vi "main.vi"() -> ()   [LabVIEW 2026]
uses:
  Controller Commands.ctl
  5a459cdc-f68a-1c45-a763-c7efc7f6e060.vi
  <vilib>/Utility/error.llb/Trim Whitespace (string).vi
  <vilib>/Utility/error.llb/Trim Whitespace One-Sided.vi
  <vilib>/Instr/_visa.llb/VISA Configure Serial Port (Instr).vi
panel:
  in  "Find Curriculum":bool
  in  "Plot to graph":bool
  in  "Reads":i32
  in  "Patameters":string[](array[string])
  in  "Command":string
  in  "Device Commands":i32(listbox)
  in  "Send Command":bool
  in  "Run Example":bool
  in  "See commands":bool
  in  "Connected Devices":i32(listbox)
  in  "Search for devices":bool
  in  "About":string="  About this app"
  in  "Status Messages":string
  in  "Exit Program":bool
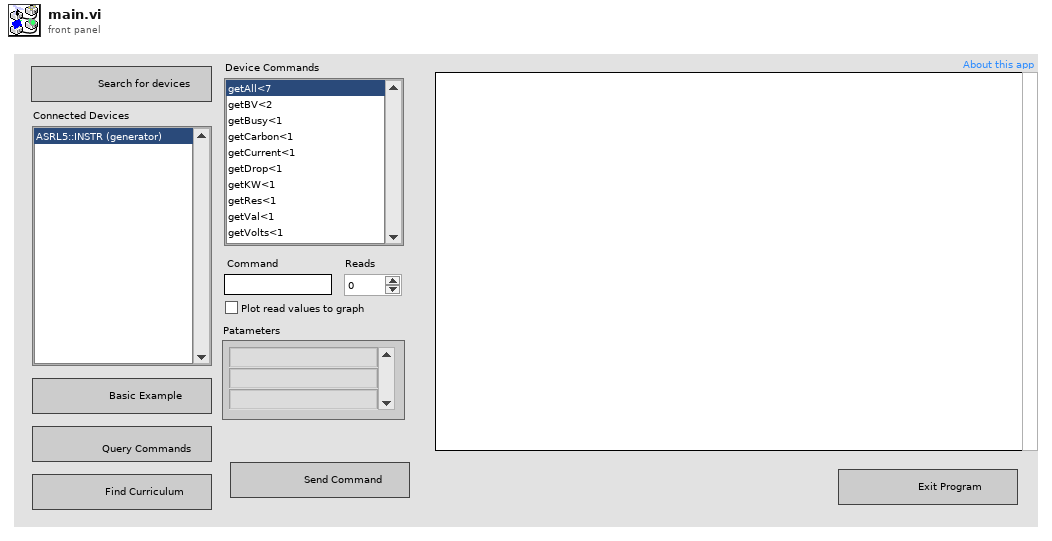
[diagram p1: front panel]
types:
  T1 = typedef "Controller Commands.ctl" = cluster{"Command":enum16{"Request Commands", "Clear all VISA aliases", "Read Reply", "Display Commands", "Command Selected", "Update UI", "Send Command", "Initialize UI", "Device Highlighted", "Run Example", "Detect Devices", "End Program", "Example Finder", "Retrieve Commands"}, "Variant":variant}
  T2 = cluster{"Connected Devices":refnum<vi>, "Device type":string[], "VISA Aliases":string[], "Status Messages":refnum<vi>, "Run Example":refnum<vi>, "See commands":refnum<vi>, "Array of VISA Resources":refnum<visa-resource-name>[], "Map of Commands":map{string, set{string}}, "Device Commands":refnum<vi>, "Command":refnum<vi>, "Patameters":refnum<vi>, "Reads":refnum<vi>, "queue for graph":refnum<queue>, "Send Command":refnum<vi>, "Find Curriculum":refnum<vi>, "appended path":path}
  T3 = enum8{"Enabled", "Disabled", "Disabled and Grayed Out"}
  T4 = enum32{"Invalid", "Standard", "Closed", "Hidden", "Minimized", "Maximized"}
  T5 = cluster{"Devices":i32, "Selected Command":string}
  T6 = enum16{"Request Commands", "Clear all VISA aliases", "Read Reply", "Display Commands", "Command Selected", "Update UI", "Send Command", "Initialize UI", "Device Highlighted", "Run Example", "Detect Devices", "End Program", "Example Finder", "Retrieve Commands"}
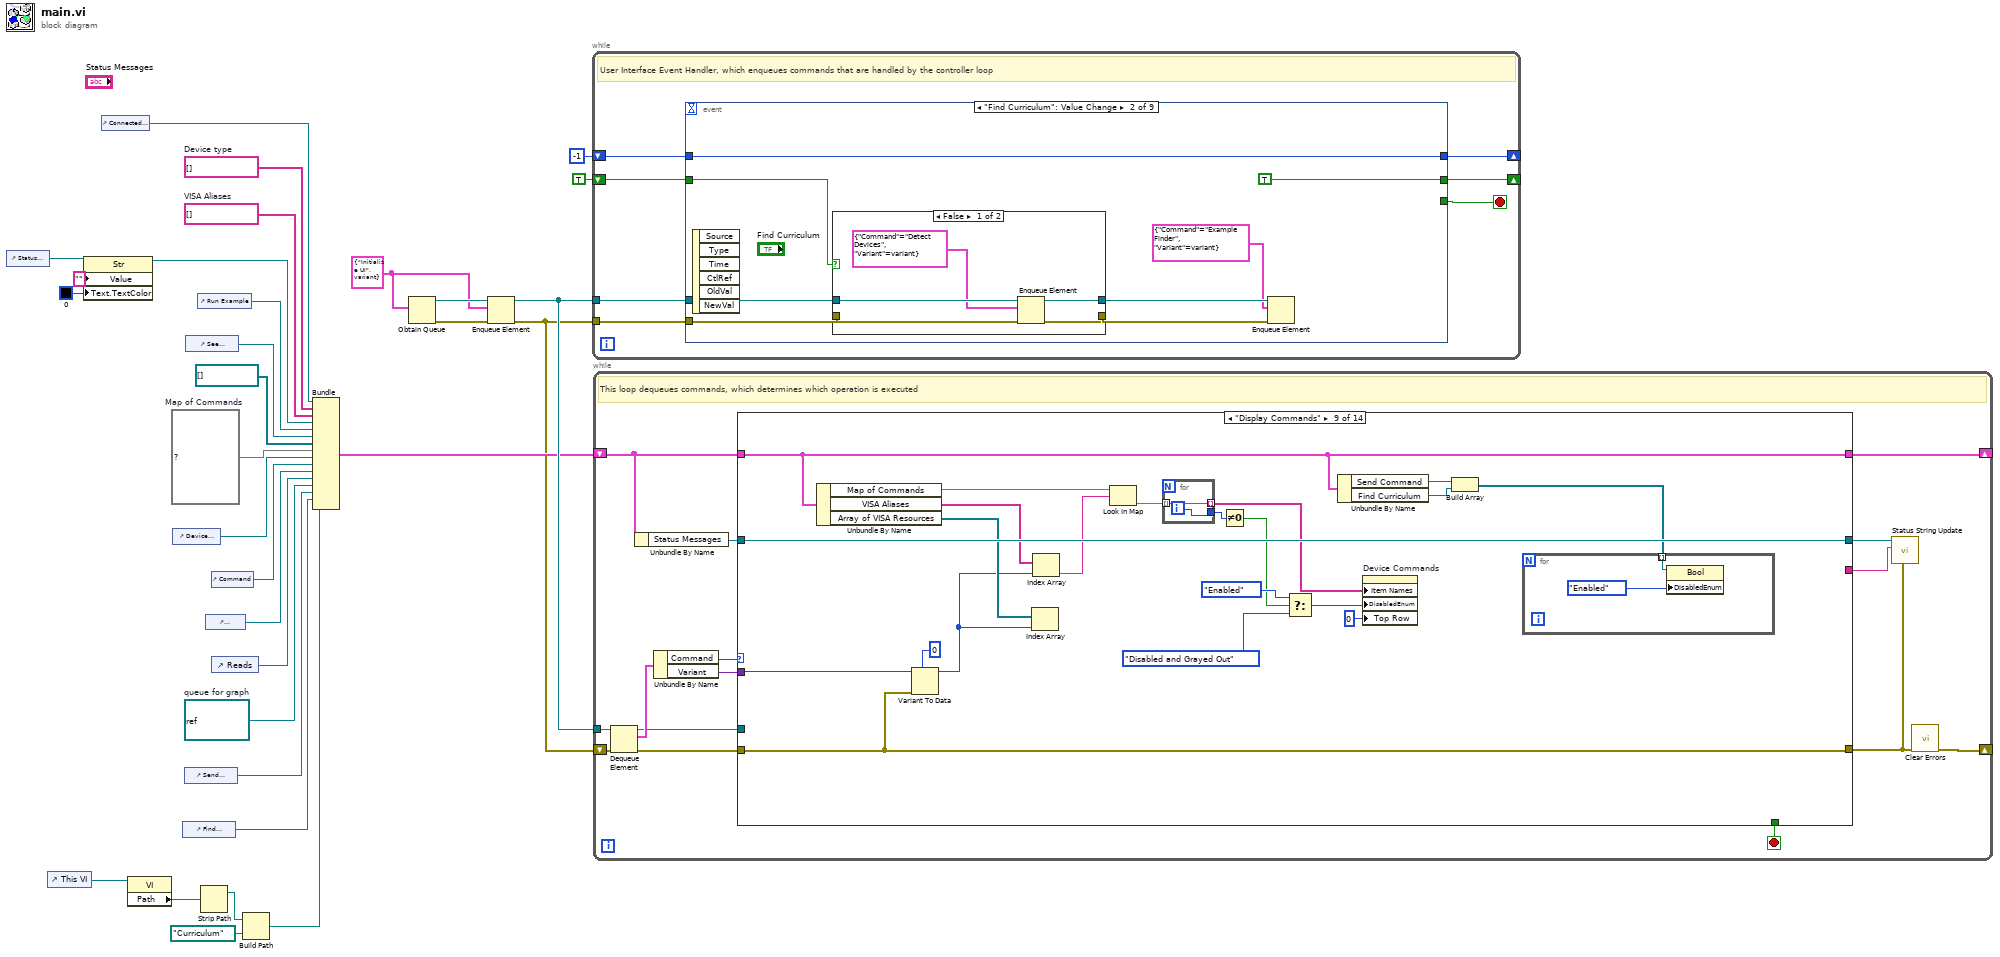
[diagram p0: block diagram]
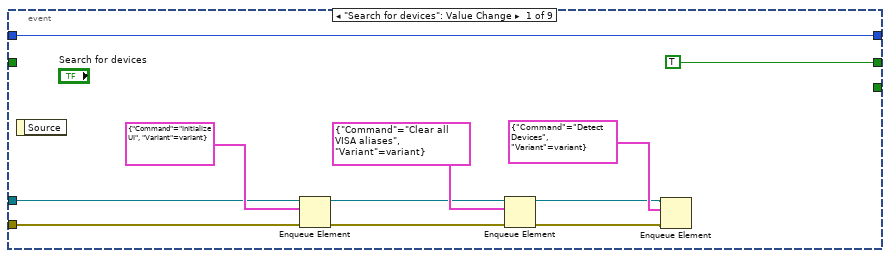
[diagram p2: hidden frame]
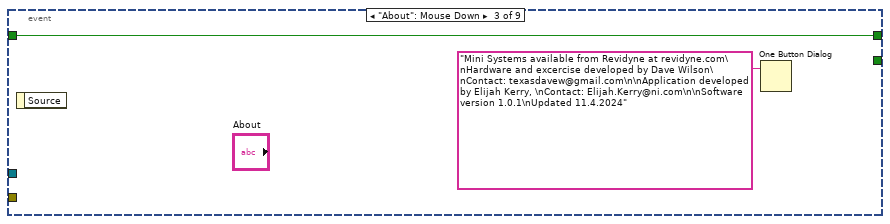
[diagram p4: hidden frame]
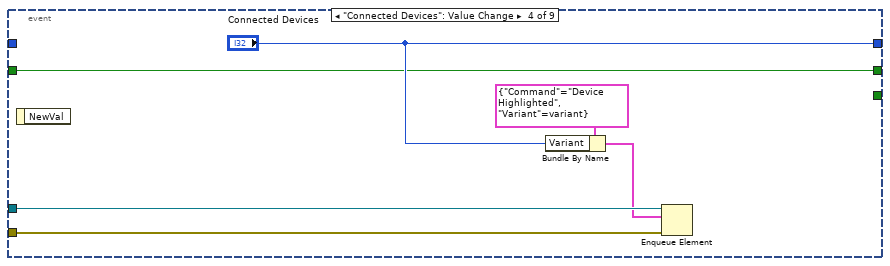
[diagram p5: hidden frame]
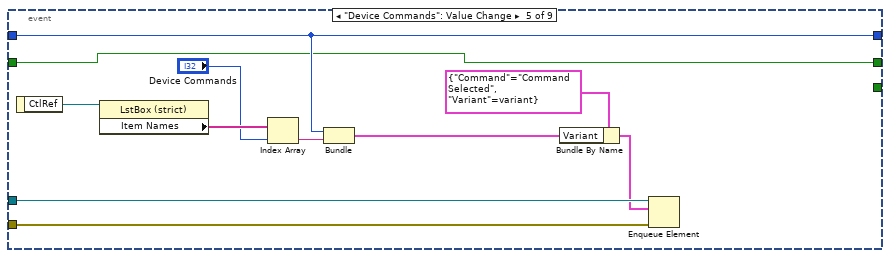
[diagram p6: hidden frame]
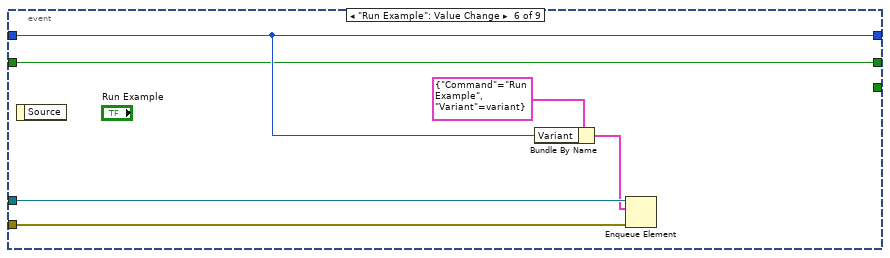
[diagram p7: hidden frame]
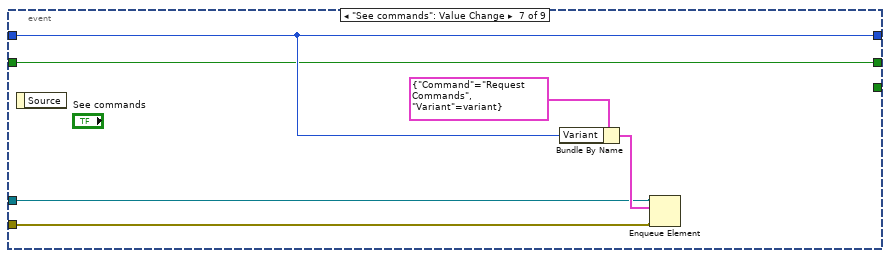
[diagram p8: hidden frame]
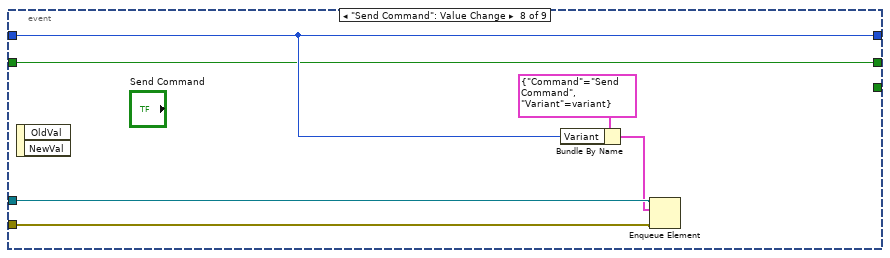
[diagram p9: hidden frame]
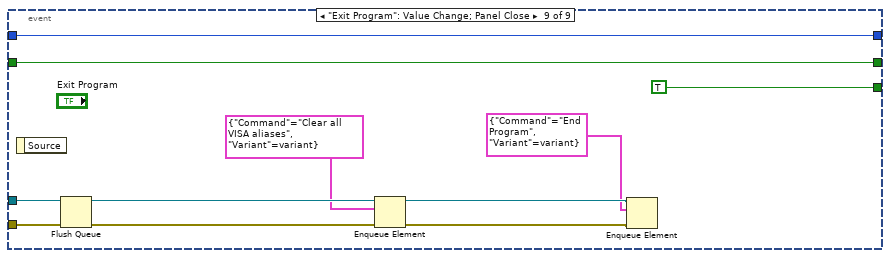
[diagram p10: hidden frame]
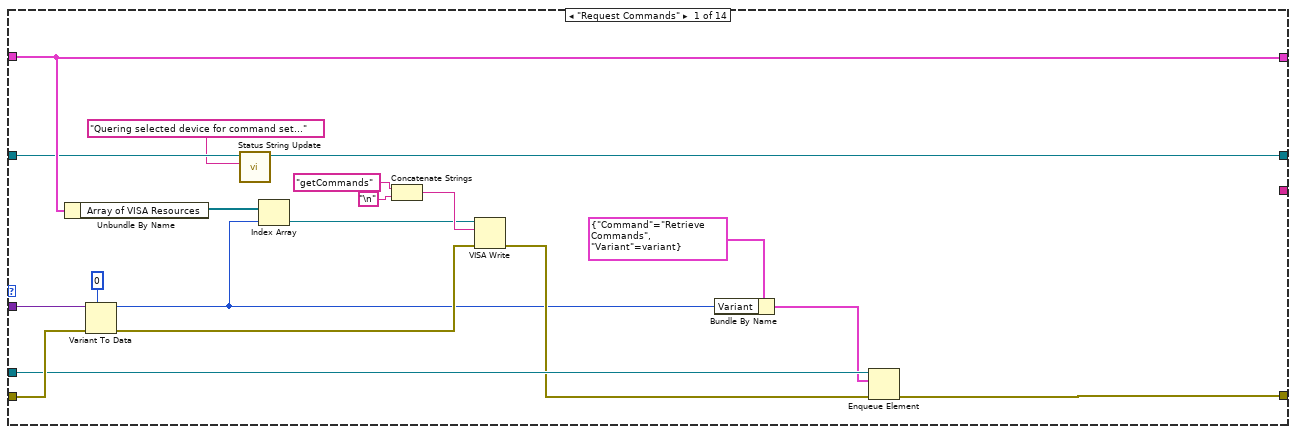
[diagram p11: hidden frame]
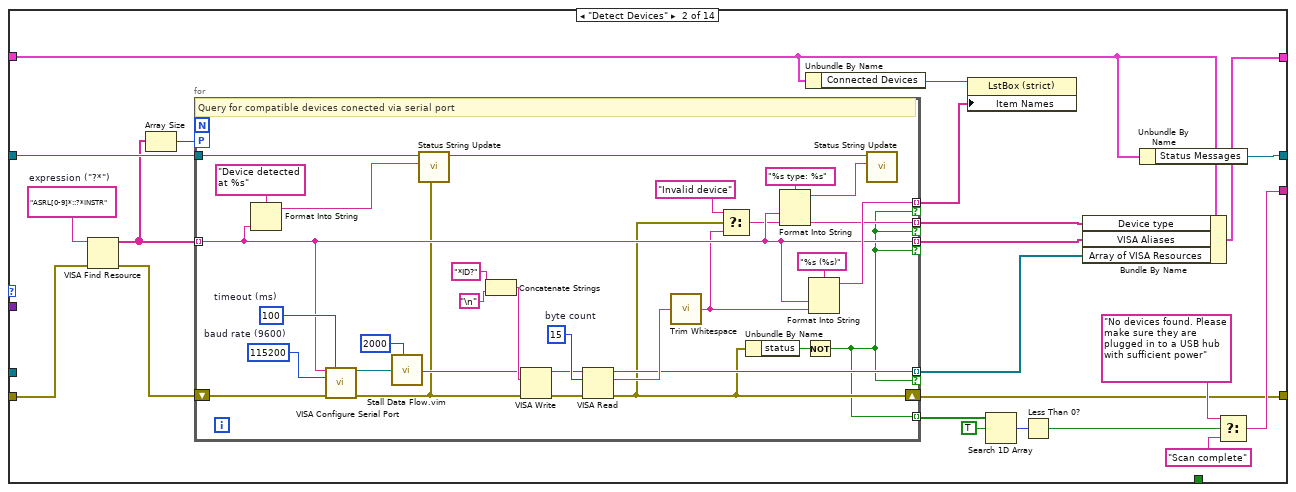
[diagram p12: hidden frame]
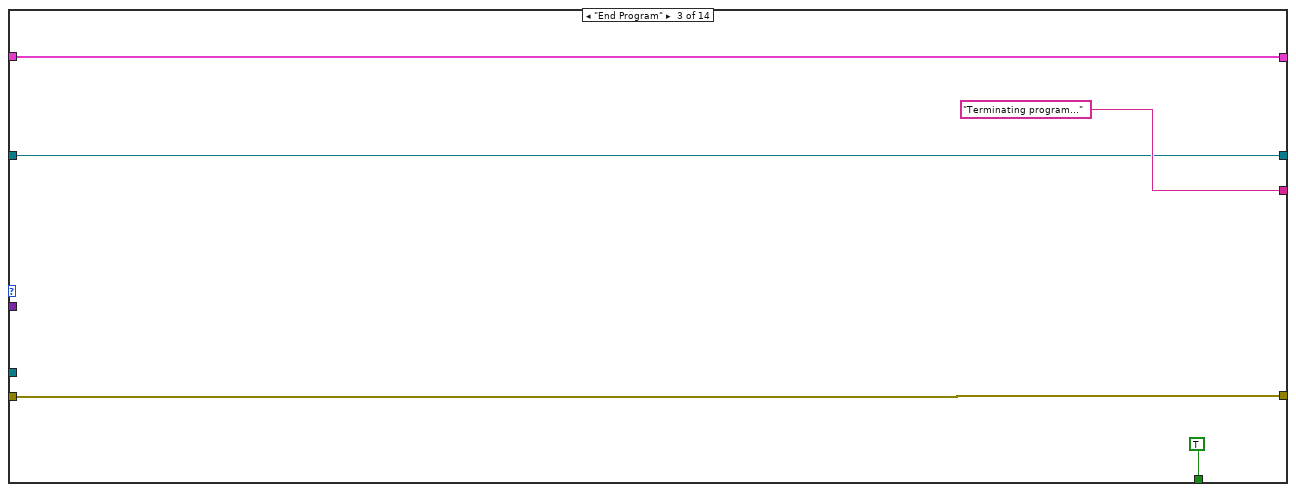
[diagram p13: hidden frame]
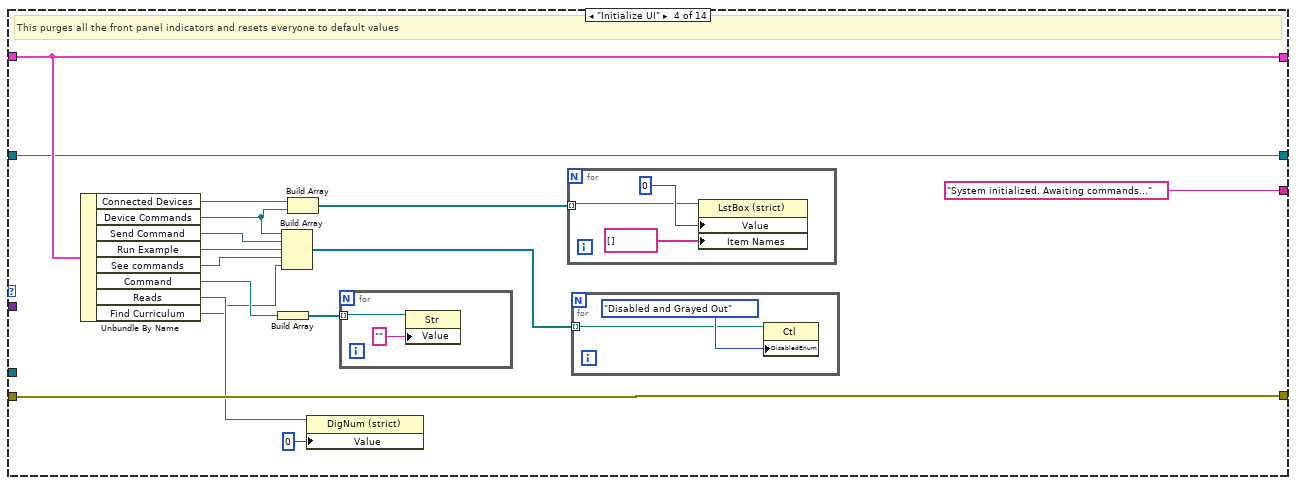
[diagram p14: hidden frame]
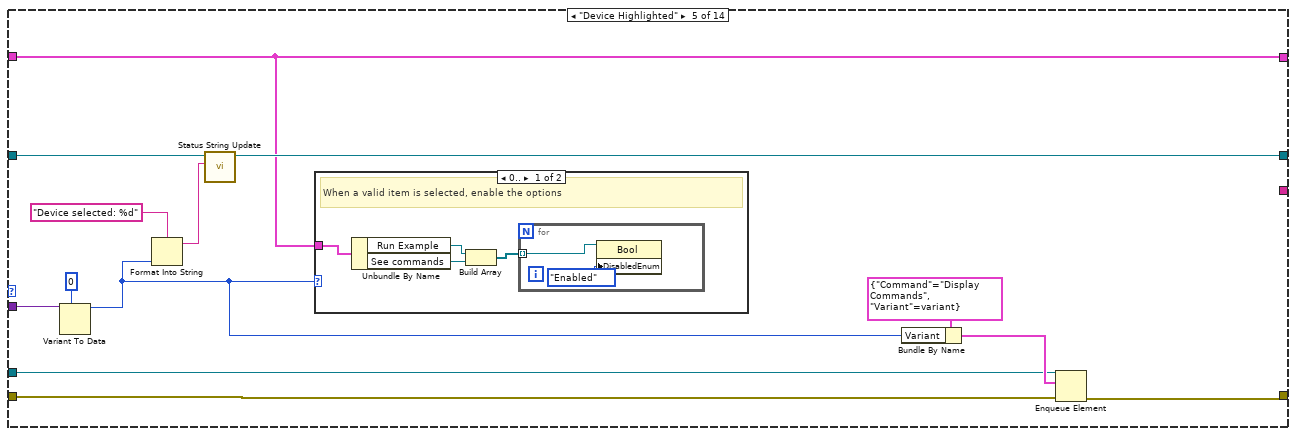
[diagram p15: hidden frame]
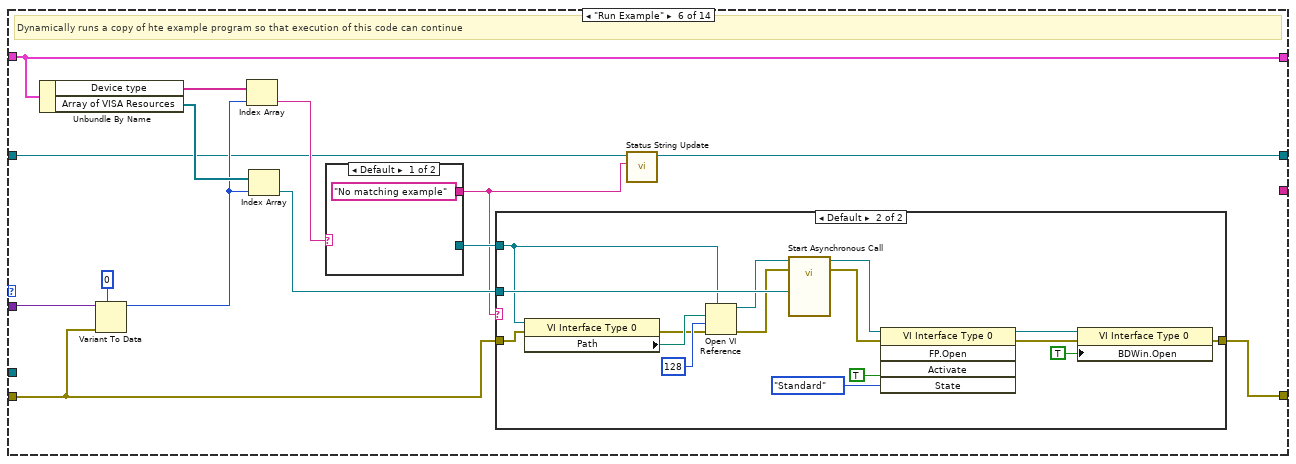
[diagram p17: hidden frame]
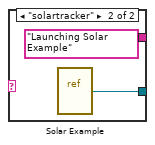
[diagram p19: hidden frame]
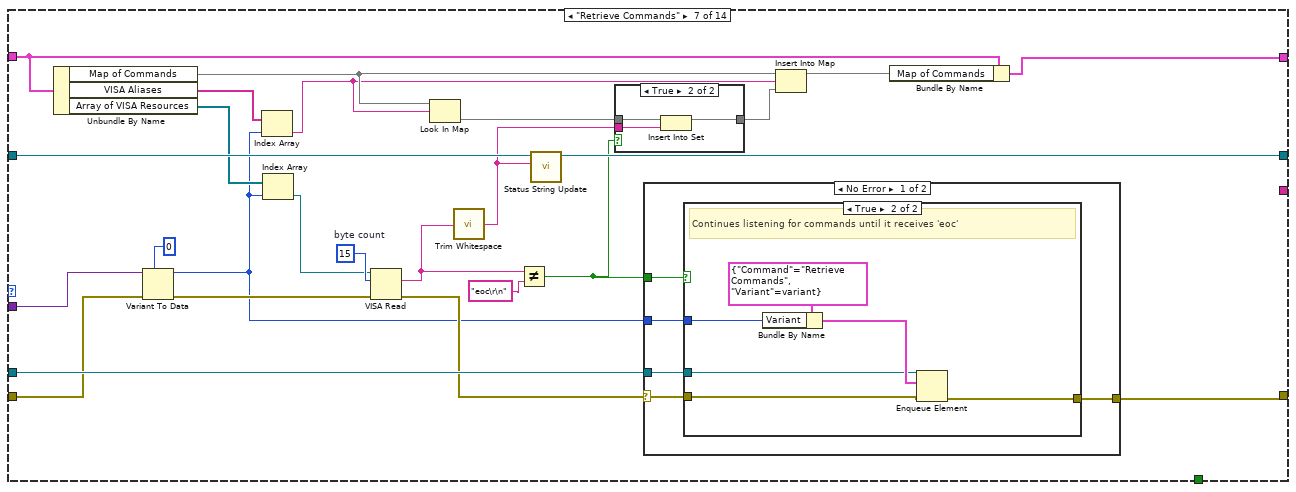
[diagram p20: hidden frame]
diagram:
  w13 = refnum<queue> refnum  # queue for graph
  w18 = map{string, set{string}} {}  # Map of Commands
  w19 = string[] []  # Device type
  w27 = string[] []  # VISA Aliases
  w29 = T1 {"Command"=enum."Initialize UI", "Variant"=variant} ("Controller Commands")
  n1 = control-ref of="Status Messages"() -> (w11:refnum<vi>)
  n2 = control-ref of="This VI"() -> (w4:refnum<vi>)
  n3 = property on="Property Node" class="Str"(reference=w11, "Value"="", "Text.TextColor"=u32 0 ("Text.Text Colors:Text Color")) -> (reference out=w10:refnum<vi>)  [unwired: 1 in, 1 out]
  n4 = control-ref of="Connected Devices"() -> (w20:refnum<vi>)
  n5 = property class="VI"(reference=w4) -> ("Path"=w5:path)  [unwired: 1 in, 2 out]
  n6 = control-ref of="Device Commands"() -> (w17:refnum<vi>)
  n7 = control-ref of="Find Curriculum"() -> (w7:refnum<vi>)
  n8 = control-ref of="Send Command"() -> (w12:refnum<vi>)
  n9 = control-ref of="See commands"() -> (w24:refnum<vi>)
  n10 = control-ref of="Run Example"() -> (w25:refnum<vi>)
  n11 = Strip Path(path=w5) -> (stripped path=w6:path)  [unwired: 1 out]
  n12 = control-ref of="Patameters"() -> (w15:refnum<vi>)
  n13 = control-ref of="Command"() -> (w16:refnum<vi>)
  n14 = control-ref of="Reads"() -> (w14:refnum<vi>)
  n15 = Build Path(base path=w6, name or relative path=path "Curriculum") -> (appended path=w2:path)
  n16 = Bundle("Connected Devices"=w20, "Device type"=w19, "VISA Aliases"=w27, "Status Messages"=w10, "Run Example"=w25, "See commands"=w24, "Array of VISA Resources"=refnum<visa-resource-name>[] [], "Map of Commands"=w18, "Device Commands"=w17, "Command"=w16, "Patameters"=w15, "Reads"=w14, "queue for graph"=w13, "Send Command"=w12, "Find Curriculum"=w7, "appended path"=w2) -> (w26:T2)  [unwired: 1 in]
  n17 = Obtain Queue(element data type=w29) -> (queue out=w31:refnum<queue>, error out=w28:errorcluster)  [unwired: 4 in, 1 out]
  n18 = Enqueue Element(queue=w31, element=w29, error in (no error)=w28) -> (queue out=w30:refnum<queue>, error out=w23:errorcluster)  [unwired: 1 in, 1 out]
  n19 = while {
    tunnel: w30 -> [w35]
    tunnel: w23 -> [w34]
    shift-right: [w37] -> _
    shift-left: -1 ("Connected Devices") -> [w36]
    shift-right: [w32] -> _
    shift-left: TRUE ("Find Curriculum") -> [w33]
    stop <- w38 stop-if-true
    # "User Interface Event Handler, which enqueues commands that are handled by the controller loop"
    n20 = event shown="[1] \"Find Curriculum\": Value Change" {
      selector: _ -> [_ _ _ _ _ _ _ _ _]
      dyn-events: _ -> [_ _ _ _ _ _ _ _ _]
      timeout: _ -> [_ _ _ _ _ _ _ _ _]
      tunnel: [_ _ _ _ _ _ _ _ TRUE] -> w38
      tunnel: w36 -> [w49 w55 _ _ w78 w88 w94 w100 w111]
      tunnel: [w49 w55 _ "Connected Devices" w78 w88 w94 w100 w111] -> w37
      tunnel: w35 -> [w44 w57 _ w69 w75 w86 w91 w98 w110]
      tunnel: w34 -> [w43 w56 _ w68 w74 w85 w90 w96 w109]
      tunnel: w33 -> [_ w54 w66 w70 w76 w87 w93 w99 w105]
      tunnel: [TRUE ("Find Curriculum") TRUE ("Find Curriculum") w66 w70 w76 w87 w93 w99 w105] -> w32
      event "Search for devices": Value Change {
        n21 = event-data() -> ()  [unwired: 1 in, 1 out]
        n22 = Enqueue Element(queue=w44, element=T1 {"Command"=enum."Initialize UI", "Variant"=variant}, error in (no error)=w43) -> (queue out=w45:refnum<queue>, error out=w46:errorcluster)  [unwired: 1 in, 1 out]
        n23 = Enqueue Element(queue=w45, element=T1 {"Command"=enum."Clear all VISA aliases", "Variant"=variant}, error in (no error)=w46) -> (queue out=w40:refnum<queue>, error out=w39:errorcluster)  [unwired: 1 in, 1 out]
        n24 = Enqueue Element(queue=w40, element=T1 {"Command"=enum."Detect Devices", "Variant"=variant}, error in (no error)=w39) -> ()  [unwired: 1 in, 3 out]
      }
      event "Find Curriculum": Value Change {
        n25 = event-data() -> ()  [unwired: 1 in, 6 out]
        n26 = case shown="False" w54 {
          tunnel: w57 -> [w62 w64]
          tunnel: [w61 w64] -> w52
          tunnel: w56 -> [w60 w63]
          tunnel: [w59 w63] -> w51
          frame False {
            n27 = Enqueue Element(queue=w62, element=T1 {"Command"=enum."Detect Devices", "Variant"=variant}, error in (no error)=w60) -> (queue out=w61:refnum<queue>, error out=w59:errorcluster)  [unwired: 1 in, 1 out]
          }
          frame True {
          }
        }
        n28 = Enqueue Element(queue=w52, element=T1 {"Command"=enum."Example Finder", "Variant"=variant}, error in (no error)=w51) -> ()  [unwired: 1 in, 3 out]
      }
      event "About": Mouse Down {
        n29 = event-data() -> ()  [unwired: 1 in, 1 out]
        n30 = One Button Dialog(message="Mini Systems available from Revidyne at revidyne.com\nHardware and excercise developed by Dave Wilson\nContact: texasdavew@gmail.com\n\nApplication developed by Elijah Kerry, \nContact: Elijah.Kerry@ni.com\n\nSoftware version 1.0.1\nUpdated 11.4.2024") -> ()  [unwired: 1 in, 1 out]
      }
      event "Connected Devices": Value Change {
        n31 = event-data() -> ()  [unwired: 1 in, 1 out]
        n32 = Bundle By Name(cluster=T1 {"Command"=enum."Device Highlighted", "Variant"=variant} ("Controller Commands"), "Variant"="Connected Devices") -> (w67:T1)
        n33 = Enqueue Element(queue=w69, element=w67, error in (no error)=w68) -> ()  [unwired: 1 in, 3 out]
      }
      event "Device Commands": Value Change {
        n34 = event-data() -> ("CtlRef"=w82:refnum<vi>)  [unwired: 1 in]
        n35 = property class="LstBox (strict)"(reference=w82) -> ("Item Names"=w81:string[])  [unwired: 1 in, 2 out]
        n36 = Index Array(array=w81, index="Device Commands") -> (element=w77:string)
        n37 = Bundle("Connected Devices"=w78, w77) -> (w79:cluster{"Connected Devices":i32, string})  [unwired: 1 in]
        n38 = Bundle By Name(cluster=T1 {"Command"=enum."Command Selected", "Variant"=variant} ("Controller Commands"), "Variant"=w79) -> (w73:T1)
        n39 = Enqueue Element(queue=w75, element=w73, error in (no error)=w74) -> ()  [unwired: 1 in, 3 out]
      }
      event "Run Example": Value Change {
        n40 = event-data() -> ()  [unwired: 1 in, 1 out]
        n41 = Bundle By Name(cluster=T1 {"Command"=enum."Run Example", "Variant"=variant} ("Controller Commands"), "Variant"=w88) -> (w84:T1)
        n42 = Enqueue Element(queue=w86, element=w84, error in (no error)=w85) -> ()  [unwired: 1 in, 3 out]
      }
      event "See commands": Value Change {
        n43 = event-data() -> ()  [unwired: 1 in, 1 out]
        n44 = Bundle By Name(cluster=T1 {"Command"=enum."Request Commands", "Variant"=variant} ("Controller Commands"), "Variant"=w94) -> (w92:T1)
        n45 = Enqueue Element(queue=w91, element=w92, error in (no error)=w90) -> ()  [unwired: 1 in, 3 out]
      }
      event "Send Command": Value Change {
        n46 = event-data() -> ()  [unwired: 1 in, 2 out]
        n47 = Bundle By Name(cluster=T1 {"Command"=enum."Send Command", "Variant"=variant} ("Controller Commands"), "Variant"=w100) -> (w97:T1)
        n48 = Enqueue Element(queue=w98, element=w97, error in (no error)=w96) -> ()  [unwired: 1 in, 3 out]
      }
      event "Exit Program": Value Change; Panel Close {
        n49 = event-data() -> ()  [unwired: 1 in, 1 out]
        n50 = Flush Queue(queue=w110, error in (no error)=w109) -> (queue out=w107:refnum<queue>, error out=w108:errorcluster)  [unwired: 1 out]
        n51 = Enqueue Element(queue=w107, element=T1 {"Command"=enum."Clear all VISA aliases", "Variant"=variant}, error in (no error)=w108) -> (queue out=w104:refnum<queue>, error out=w103:errorcluster)  [unwired: 1 in, 1 out]
        n52 = Enqueue Element(queue=w104, element=T1 {"Command"=enum."End Program", "Variant"=variant}, error in (no error)=w103) -> ()  [unwired: 1 in, 3 out]
      }
    }
  }
  n53 = while {
    shift-right: [w122] -> _
    shift-left: w26 -> [w120]
    tunnel: w30 -> [w127]
    shift-right: [w115] -> _
    shift-left: w23 -> [w124]
    stop <- w116 stop-if-true
    # "This loop dequeues commands, which determines which operation is executed"
    n54 = Dequeue Element(queue=w127, error in (no error)=w124) -> (queue out=w114:refnum<queue>, element=w126:T1, error out=w123:errorcluster)  [unwired: 1 in, 1 out]
    n55 = Unbundle By Name(w120) -> ("Status Messages"=w119:refnum<vi>)
    n56 = Unbundle By Name(w126) -> ("Command"=w125:T6, "Variant"=w117:variant)
    n57 = case shown="\"Display Commands\"" w125 {
      tunnel: [_ _ TRUE _ _ _ _ _ _ _ _ _ _ _] -> w116
      tunnel: w120 -> [w144 w149 w200 w219 w235 w255 w289 w329 w334 w361 w410 w448 w469 w485]
      tunnel: w123 -> [w134 w167 w199 w216 w230 w251 w298 w327 w346 w376 w433 w445 w466 w479]
      tunnel: [w144 w165 w200 w219 w235 w255 w287 w329 w334 w360 w410 w448 w469 w485] -> w122
      tunnel: [_ w151 "Terminating program..." ("Value") "System initialized. Awaiting commands..." ("Value") _ _ _ _ _ _ _ _ "VISA devices closed" ("Value") _] -> w121
      tunnel: w119 -> [w138 w162 w201 w217 w239 w248 w302 w328 w350 w371 w417 w447 w465 w487]
      tunnel: [w136 w148 w201 w217 w238 w247 w283 w328 w350 w356 w416 w437 w464 w480] -> w118
      tunnel: w117 -> [w145 _ _ _ w234 w257 w303 _ w348 w377 w434 w446 _ _]
      tunnel: [w131 w150 w199 w216 w228 w249 w301 w327 w346 w358 w433 w439 w462 w473] -> w113
      tunnel: w114 -> [w133 _ _ _ w229 _ w300 _ _ w364 _ _ _ _]
      frame "Request Commands" {
        n58 = Unbundle By Name(w144) -> ("Array of VISA Resources"=w143:refnum<visa-resource-name>[])
        n59 = Variant To Data(error in=w134, type=0 ("input 1"), Variant=w145) -> (data=w128:i32, error out=w135:errorcluster)
        n60 = call "Status String Update.vi"("Value"="Quering selected device for command set...", "String reference in"=w138) -> ("STring reference out"=w136:refnum<vi>)  [unwired: 9 in]
        n61 = Index Array(array=w143, index=w128) -> (element=w139:refnum<visa-resource-name>)
        n62 = Concatenate Strings("getCommands", "\n") -> (w141:string)
        n63 = VISA Write(VISA resource name=w139, write buffer=w141, error in (no error)=w135) -> (error out=w132:errorcluster)  [unwired: 2 out]
        n64 = Bundle By Name(cluster=T1 {"Command"=enum."Retrieve Commands", "Variant"=variant}, "Variant"=w128) -> (w129:T1)
        n65 = Enqueue Element(queue=w133, element=w129, error in (no error)=w132) -> (error out=w131:errorcluster)  [unwired: 1 in, 2 out]
      }
      frame "Detect Devices" {
        w168 = "ASRL[0-9]*::?*INSTR"  # expression ("?*")
        n66 = VISA Find Resource(8:w167, 11:w168) -> (0:w158:errorcluster, 3:w159:string[])  [unwired: 1 in, 1 out]
        n67 = Array Size(array=w159) -> (size(s)=w147:i32)
        n68 = for {
          tunnel: w159 -> [w184] mode=indexing
          tunnel: [w193] -> w163 mode=indexing if=w170
          tunnel: [w184] -> w166 mode=indexing if=w170
          tunnel: w162 -> [w192]
          tunnel: [w182] -> w161 mode=indexing if=w170
          tunnel: [w181] -> w160 mode=indexing if=w170
          workers-P: w147 -> [_]
          shift-right: [w171] -> w150
          shift-left: w158 -> [w178]
          tunnel: [w170] -> w157 mode=indexing
          w196 = u32 15  # byte count
          w198 = u32 115200  # baud rate (9600)
          w197 = u32 100  # timeout (ms)
          # "Query for compatible devices conected via serial port"
          n69 = Format Into String(format string="Device detected at %s", w184) -> (resulting string=w185:string)  [unwired: 2 in, 1 out]
          n70 = call-poly "VISA Configure Serial Port"("VISA resource name"=w184, "timeout (10sec)"=w197, "baud rate (9600)"=w198, "error in (no error)"=w178) -> ("VISA resource name out"=w174:refnum<visa-resource-name>, "error out"=w169:errorcluster)  [unwired: 10 in]
          n71 = call "Stall Data Flow.vim"("value in"=w174, "milliseconds to wait"=u32 2000) -> ("value out"=w173:refnum<visa-resource-name>)  [unwired: 1 out]
          n72 = call "Status String Update.vi"("error in (no error)"=w169, "Value"=w185, "String reference in"=w192) -> ("STring reference out"=w188:refnum<vi>)  [unwired: 8 in]
          n73 = Concatenate Strings("*ID?", "\n") -> (w177:string)
          n74 = VISA Write(VISA resource name=w173, write buffer=w177, error in (no error)=w169) -> (VISA resource name out=w179:refnum<visa-resource-name>, error out=w180:errorcluster)  [unwired: 1 out]
          n75 = VISA Read(VISA resource name=w179, byte count=w196, error in (no error)=w180) -> (VISA resource name out=w182:refnum<visa-resource-name>, read buffer=w186:string, error out=w171:errorcluster)  [unwired: 1 out]
          n76 = call-poly <vilib>:"Trim Whitespace.vi"("string"=w186) -> ("trimmed string"=w183:string)  [unwired: 1 in]
          n77 = Select(t="Invalid device" ("f"), s=w171, f=w183) -> (s? t:f=w181:string)
          n78 = Unbundle By Name(w171) -> ("status"=w195:bool)
          n79 = Format Into String(format string="%s type: %s", w184, w181) -> (resulting string=w189:string)  [unwired: 2 in, 1 out]
          n80 = Not(x=w195) -> (.not. x?=w170:bool)
          n81 = Format Into String(format string="%s (%s)" ("initial string"), w184, w183) -> (resulting string=w193:string)  [unwired: 2 in, 1 out]
          n82 = call "Status String Update.vi"("Value"=w189, "String reference in"=w188) -> ()  [unwired: 9 in, 1 out]
        }
        n83 = Unbundle By Name(w149) -> ("Connected Devices"=w164:refnum<vi>)
        n84 = property class="LstBox (strict)"(reference=w164, "Item Names"=w163) -> ()  [unwired: 1 in, 2 out]
        n85 = Search 1D Array(1D array=w157, element=TRUE) -> (index of element=w155:i32)  [unwired: 1 in]
        n86 = Less Than 0?(x=w155) -> (x < 0?=w154:bool)
        n87 = Bundle By Name(cluster=w149, "Device type"=w160, "VISA Aliases"=w166, "Array of VISA Resources"=w161) -> (w165:T2)
        n88 = Unbundle By Name(w149) -> ("Status Messages"=w148:refnum<vi>)
        n89 = Select(t="No devices found. Please make sure they are plugged in to a USB hub with sufficient power" ("Value"), s=w154, f="Scan complete" ("Value")) -> (s? t:f=w151:string)
      }
      frame "End Program" {
      }
      frame "Initialize UI" {
        # "This purges all the front panel indicators and resets everyone to default values"
        n90 = Unbundle By Name(w219) -> ("Connected Devices"=w208:refnum<vi>, "Device Commands"=w206:refnum<vi>, "Send Command"=w205:refnum<vi>, "Run Example"=w214:refnum<vi>, "See commands"=w215:refnum<vi>, "Command"=w212:refnum<vi>, "Reads"=w210:refnum<vi>, "Find Curriculum"=w204:refnum<vi>)
        n91 = Build Array(w212) -> (w211:refnum<vi>[])
        n92 = Build Array(w206, w205, w214, w215, w204) -> (w213:refnum<vi>[])
        n93 = Build Array(w208, w206) -> (w207:refnum<vi>[])
        n94 = property class="DigNum (strict)"(reference=w210, "Value"=0) -> ()  [unwired: 1 in, 2 out]
        n95 = for {
          tunnel: w211 -> [w223] mode=indexing
          n96 = property class="Str"(reference=w223, "Value"="") -> ()  [unwired: 1 in, 2 out]
        }
        n97 = for {
          tunnel: w207 -> [w220] mode=indexing
          n98 = property class="LstBox (strict)"(reference=w220, "Value"=0, "Item Names"=string[] []) -> ()  [unwired: 1 in, 2 out]
        }
        n99 = for {
          tunnel: w213 -> [w225] mode=indexing
          n100 = property class="Ctl"(reference=w225, "DisabledEnum"=T3."Disabled and Grayed Out" ("Disabled")) -> ()  [unwired: 1 in, 2 out]
        }
      }
      frame "Device Highlighted" {
        n101 = Variant To Data(type=0 ("input 1"), Variant=w234) -> (data=w227:i32)  [unwired: 1 in, 1 out]
        n102 = Format Into String(format string="Device selected: %d", w227) -> (resulting string=w236:string)  [unwired: 2 in, 1 out]
        n103 = call "Status String Update.vi"("Value"=w236, "String reference in"=w239) -> ("STring reference out"=w238:refnum<vi>)  [unwired: 9 in]
        n104 = case shown="0.." w227 {
          tunnel: w235 -> [w243 _]
          frame 0.. {
            # "When a valid item is selected, enable the options"
            n105 = Unbundle By Name(w243) -> ("Run Example"=w242:refnum<vi>, "See commands"=w240:refnum<vi>)
            n106 = Build Array(w242, w240) -> (w241:refnum<vi>[])
            n107 = for {
              tunnel: w241 -> [w244] mode=indexing
              n108 = property class="Bool"(reference=w244, "DisabledEnum"=T3."Enabled" ("Disabled")) -> ()  [unwired: 1 in, 2 out]
            }
          }
          frame Default {
          }
        }
        n109 = Bundle By Name(cluster=T1 {"Command"=enum."Display Commands", "Variant"=variant}, "Variant"=w227) -> (w231:T1)
        n110 = Enqueue Element(queue=w229, element=w231, error in (no error)=w230) -> (error out=w228:errorcluster)  [unwired: 1 in, 2 out]
      }
      frame "Run Example" {
        # "Dynamically runs a copy of hte example program so that execution of this code can continue"
        n111 = Unbundle By Name(w255) -> ("Device type"=w252:string[], "Array of VISA Resources"=w258:refnum<visa-resource-name>[])
        n112 = Variant To Data(error in=w251, type=0 ("input 1"), Variant=w257) -> (data=w254:i32)  [unwired: 1 out]
        n113 = Index Array(array=w252, index=w254) -> (element=w253:string)
        n114 = Index Array(array=w258, index=w254) -> (element=w256:refnum<visa-resource-name>)
        n115 = case shown="Default" w253 {
          tunnel: [_ w279] -> w250
          tunnel: ["No matching example" ("Value") "Launching Solar Example" ("Value")] -> w246
          frame Default {
          }
          frame "solartracker" {
            n116 = vi-ref "Solar Example.vi"() -> (w279:refnum<vi>)
          }
        }
        n117 = case shown="Default" w246 {
          tunnel: w256 -> [_ w276]
          tunnel: w251 -> [w260 w268]
          tunnel: w250 -> [_ w265]
          tunnel: [w260 w262] -> w249
          frame "No matching example" {
          }
          frame Default {
            n118 = property class="VI Interface Type 0"(reference=w265, error in=w268) -> (error out=w267:errorcluster, "Path"=w272:path)  [unwired: 1 out]
            n119 = Open VI Reference(type specifier VI Refnum (for type only)=w265, vi path=w272, options=128, error in (no error)=w267) -> (vi reference=w275:refnum<vi>, error out=w273:errorcluster)  [unwired: 2 in]
            n120 = call-by-ref "Start Asynchronous Call"(reference=w275, error in=w273, "VISA resource name 2"=w276) -> (reference out=w266:refnum<vi>, error out=w269:errorcluster)  [unwired: 11 in]
            n121 = invoke class="VI Interface Type 0" method="FP.Open"(reference=w266, error in=w269, "Activate"=TRUE ("Activate?"), "State"=T4."Standard") -> (reference out=w264:refnum<vi>, error out=w263:errorcluster)  [unwired: 1 in, 3 out]
            n122 = property class="VI Interface Type 0"(reference=w264, error in=w263, "BDWin.Open"=TRUE ("Block Diagram Window:Open")) -> (error out=w262:errorcluster)  [unwired: 1 out]
          }
        }
        n123 = call "Status String Update.vi"("Value"=w246, "String reference in"=w248) -> ("STring reference out"=w247:refnum<vi>)  [unwired: 9 in]
      }
      frame "Retrieve Commands" {
        w304 = u32 15  # byte count
        n124 = Unbundle By Name(w289) -> ("Map of Commands"=w286:map{string, set{string}}, "VISA Aliases"=w292:string[], "Array of VISA Resources"=w295:refnum<visa-resource-name>[])
        n125 = Variant To Data(error in=w298, type=0 ("input 1"), Variant=w303) -> (data=w291:i32, error out=w297:errorcluster)
        n126 = Index Array(array=w292, index=w291) -> (element=w285:string)
        n127 = Index Array(array=w295, index=w291) -> (element=w294:refnum<visa-resource-name>)
        n128 = VISA Read(VISA resource name=w294, byte count=w304, error in (no error)=w297) -> (read buffer=w282:string, error out=w299:errorcluster)  [unwired: 2 out]
        n129 = Look In Map(map=w286, key=w285) -> (value=w284:set{string})  [unwired: 1 in, 1 out]
        n130 = call-poly <vilib>:"Trim Whitespace.vi"("string"=w282) -> ("trimmed string"=w293:string)  [unwired: 1 in]
        n131 = Not Equal?(x=w282, y="eoc\r\n" ("read buffer")) -> (x != y?=w280:bool)
        n132 = call "Status String Update.vi"("Value"=w293, "String reference in"=w302) -> ("STring reference out"=w283:refnum<vi>)  [unwired: 9 in]
        n133 = case shown="True" w280 {
          tunnel: w293 -> [_ w308]
          tunnel: [w305 w307] -> w290
          tunnel: w284 -> [w305 w306]
          frame False {
          }
          frame True {
            n134 = Insert Into Set(10:w308, 11:w306) -> (3:w307:set{string})  [unwired: 1 out]
          }
        }
        n135 = case shown="No Error" w299 {
          selector: w299 -> [w309 w326]
          tunnel: w291 -> [w313 _]
          tunnel: [w312 w326] -> w301
          tunnel: w280 -> [w311 _]
          tunnel: w300 -> [w310 _]
          frame No Error {
            n136 = case shown="True" w311 {
              tunnel: w313 -> [w317 w323]
              tunnel: w309 -> [w315 w322]
              tunnel: [w314 w321] -> w312
              tunnel: w310 -> [w316 w320]
              frame False {
                n137 = Bundle By Name(cluster=T1 {"Command"=enum."Display Commands", "Variant"=variant}, "Variant"=w317) -> (w318:T1)
                n138 = Enqueue Element(queue=w316, element=w318, error in (no error)=w315) -> (error out=w314:errorcluster)  [unwired: 1 in, 2 out]
              }
              frame True {
                # "Continues listening for commands until it receives 'eoc'"
                n139 = Bundle By Name(cluster=T1 {"Command"=enum."Retrieve Commands", "Variant"=variant}, "Variant"=w323) -> (w324:T1)
                n140 = Enqueue Element(queue=w320, element=w324, error in (no error)=w322) -> (error out=w321:errorcluster)  [unwired: 1 in, 2 out]
              }
            }
          }
          frame Error {
          }
        }
        n141 = Insert Into Map(map in=w286, key=w285, value=w290) -> (map out=w288:map{string, set{string}})  [unwired: 2 out]
        n142 = Bundle By Name(cluster=w289, "Map of Commands"=w288) -> (w287:T2)
      }
      frame "Update UI" {
      }
      frame "Display Commands" {
        n143 = Unbundle By Name(w334) -> ("Map of Commands"=w345:map{string, set{string}}, "VISA Aliases"=w347:string[], "Array of VISA Resources"=w344:refnum<visa-resource-name>[])
        n144 = Variant To Data(error in=w346, type=0 ("input 1"), Variant=w348) -> (data=w343:i32)  [unwired: 1 out]
        n145 = Index Array(array=w344, index=w343) -> ()  [unwired: 1 out]
        n146 = Index Array(array=w347, index=w343) -> (element=w342:string)
        n147 = Look In Map(map=w345, key=w342) -> (value=w341:set{string})  [unwired: 1 in, 1 out]
        n148 = for {
          tunnel: [w354] -> w340 mode=indexing
          tunnel: w341 -> [w354] mode=indexing
          tunnel: [w353] -> w336
          i -> [w353]
        }
        n149 = Not Equal To 0?(x=w336) -> (x != 0?=w335:bool)
        n150 = Select(t=T3."Enabled" ("Disabled"), s=w335, f=T3."Disabled and Grayed Out" ("Disabled")) -> (s? t:f=w337:T3)
        n151 = Unbundle By Name(w334) -> ("Send Command"=w332:refnum<vi>, "Find Curriculum"=w333:refnum<vi>)
        n152 = property on="Device Commands" class="LstBox (strict)"("Item Names"=w340, "DisabledEnum"=w337, "Top Row"=0 ("Device Commands")) -> ()  [unwired: 2 in, 2 out]
        n153 = Build Array(w332, w333) -> (w331:refnum<vi>[])
        n154 = for {
          tunnel: w331 -> [w351] mode=indexing
          n155 = property class="Bool"(reference=w351, "DisabledEnum"=T3."Enabled" ("Disabled")) -> ()  [unwired: 1 in, 2 out]
        }
      }
      frame "Send Command" {
        n156 = Unbundle By Name(w361) -> ("Array of VISA Resources"=w374:refnum<visa-resource-name>[])
        n157 = Variant To Data(error in=w376, type=0 ("input 1"), Variant=w377) -> (data=w362:i32, error out=w368:errorcluster)
        n158 = for {
          tunnel: "Patameters" -> [w407] mode=indexing
          shift-right: [w406] -> w365
          shift-left: "Command" -> [w405]
          n159 = Concatenate Strings(w405, " " ("string"), w407) -> (w406:string)
        }
        n160 = Index Array(array=w374, index=w362) -> (element=w373:refnum<visa-resource-name>)
        n161 = Format Into String(format string="Sending command '%s'", w365) -> (resulting string=w369:string)  [unwired: 2 in, 1 out]
        n162 = Concatenate Strings(w365, "\n") -> (w372:string)
        n163 = call "Status String Update.vi"("Value"=w369, "String reference in"=w371) -> ("STring reference out"=w357:refnum<vi>)  [unwired: 9 in]
        n164 = VISA Write(VISA resource name=w373, write buffer=w372, error in (no error)=w368) -> (error out=w359:errorcluster)  [unwired: 2 out]
        n165 = for {
          N: "Reads" -> [_]
          tunnel: w364 -> [w401]
          shift-right: [w399] -> _
          shift-left: w359 -> [w400]
          tunnel: w362 -> [w397]
          tunnel: "Plot to graph" -> [w396]
          n166 = Bundle("Plot to graph"=w396, "input 1"=w397) -> (w398:cluster{"Plot to graph":bool, "input 1":i32})  [unwired: 1 in]
          n167 = Bundle By Name(cluster=T1 {"Command"=enum."Read Reply", "Variant"=variant}, "Variant"=w398) -> (w402:T1)
          n168 = Enqueue Element(queue=w401, element=w402, error in (no error)=w400) -> (error out=w399:errorcluster)  [unwired: 1 in, 2 out]
        }
        n169 = case shown="True" "Plot to graph" {
          tunnel: w361 -> [w379 w394]
          tunnel: [w379 w393] -> w360
          tunnel: w359 -> [w380 w392]
          tunnel: [w380 w391] -> w358
          tunnel: w357 -> [w381 w390]
          tunnel: [w381 w389] -> w356
          frame False {
          }
          frame True {
            n170 = Obtain Queue(element data type=0.0, error in (no error)=w392) -> (queue out=w383:refnum<queue>, error out=w391:errorcluster)  [unwired: 3 in, 1 out]
            n171 = vi-ref "Graph Popup.vi"() -> (w385:refnum<vi>)
            n172 = property class="VI Interface Type 1"(reference=w385) -> ("Path"=w387:path)  [unwired: 1 in, 2 out]
            n173 = Bundle By Name(cluster=w394, "queue for graph"=w383) -> (w393:T2)
            n174 = Open VI Reference(type specifier VI Refnum (for type only)=w385, vi path=w387, options=128) -> (vi reference=w384:refnum<vi>, error out=w382:errorcluster)  [unwired: 3 in]
            n175 = call "Status String Update.vi"("error in (no error)"=w382, "Value"="Launching the graph", "String reference in"=w390) -> ("STring reference out"=w389:refnum<vi>)  [unwired: 8 in]
            n176 = call-by-ref "Start Asynchronous Call"(reference=w384, error in=w382, "Queue for data"=w383) -> ()  [unwired: 11 in, 2 out]
          }
        }
      }
      frame "Command Selected" {
        # "Finds number of inputs"
        # "Finds number of outputs"
        # "Determines if a command has been selected and populates the parameters and number of reads"
        n177 = Variant To Data(error in=w433, type=T5 {"Devices"=0, "Selected Command"=""} ("output cluster"), Variant=w434) -> (data=w431:T5)  [unwired: 1 out]
        n178 = Unbundle(w431) -> ("Selected Command"=w428:string)  [unwired: 1 out]
        n179 = Match Pattern(string=w428, regular expression="<") -> (before substring=w427:string, after substring=w412:string, offset past match=w425:i32)  [unwired: 1 in, 1 out]
        n180 = Unbundle By Name(w410) -> ("Patameters"=w421:refnum<vi>, "Command"=w430:refnum<vi>)
        n181 = Not Equal?(x=w425, y=-1) -> ()  [unwired: 1 out]
        n182 = Match Pattern(string=w427, regular expression=">") -> (before substring=w411:string, after substring=w420:string, offset past match=w422:i32)  [unwired: 1 in, 1 out]
        n183 = property class="Str"(reference=w430, "Value"=w411) -> ()  [unwired: 1 in, 2 out]
        n184 = Not Equal?(x=w422, y=-1) -> ()  [unwired: 1 out]
        n185 = Decimal String To Number(string=w420) -> (number=w413:i32)  [unwired: 2 in, 1 out]
        n186 = Decimal String To Number(string=w412) -> (number=w408:i32)  [unwired: 2 in, 1 out]
        n187 = Initialize Array("0", w413) -> (w419:string[])
        n188 = property class="Arr (strict)"(reference=w421, "Value"=w419) -> ()  [unwired: 1 in, 2 out]
        n189 = Format Into String(format string="Command '%s' selected. It expects %d inputs and returns %d ouputs", w411, w413, w408) -> (resulting string=w414:string)  [unwired: 2 in, 1 out]
        n190 = call "Status String Update.vi"("Value"=w414, "String reference in"=w417) -> ("STring reference out"=w416:refnum<vi>)  [unwired: 9 in]
        n191 = Unbundle By Name(w410) -> ("Reads"=w409:refnum<vi>)
        n192 = property class="DigNum (strict)"(reference=w409, "Value"=w408) -> ()  [unwired: 1 in, 2 out]
      }
      frame "Read Reply" {
        w453 = u32 15  # byte count
        n193 = Unbundle By Name(w448) -> ("queue for graph"=w436:refnum<queue>, "Array of VISA Resources"=w451:refnum<visa-resource-name>[])
        n194 = Variant To Data(error in=w445, type=cluster{"Plot to graph":bool, "input 1":i32} {"Plot to graph"=FALSE, "input 1"=0} ("output cluster"), Variant=w446) -> (data=w443:cluster{"Plot to graph":bool, "input 1":i32}, error out=w452:errorcluster)
        n195 = Unbundle(w443) -> ("Plot to graph"=w441:bool, "input 1"=w442:i32)
        n196 = Index Array(array=w451, index=w442) -> (element=w450:refnum<visa-resource-name>)
        n197 = VISA Read(VISA resource name=w450, byte count=w453, error in (no error)=w452) -> (read buffer=w435:string, error out=w438:errorcluster)  [unwired: 2 out]
        n198 = call-poly <vilib>:"Trim Whitespace.vi"("string"=w435) -> ("trimmed string"=w449:string)  [unwired: 1 in]
        n199 = call "Status String Update.vi"("Value"=w449, "String reference in"=w447) -> ("STring reference out"=w440:refnum<vi>)  [unwired: 9 in]
        n200 = case shown="True" w441 {
          tunnel: w440 -> [w455 w461]
          tunnel: [w454 w456] -> w439
          tunnel: w438 -> [w454 w457]
          tunnel: [w455 w461] -> w437
          tunnel: w436 -> [_ w460]
          tunnel: w435 -> [_ w459]
          frame False {
          }
          frame True {
            n201 = Fract/Exp String To Number(string=w459) -> (number=w458:dbl)  [unwired: 3 in, 1 out]
            n202 = Enqueue Element(queue=w460, element=w458, error in (no error)=w457) -> (error out=w456:errorcluster)  [unwired: 1 in, 2 out]
          }
        }
      }
      frame "Clear all VISA aliases" {
        n203 = Unbundle By Name(w469) -> ("Array of VISA Resources"=w467:refnum<visa-resource-name>[])
        n204 = call "Status String Update.vi"("error in (no error)"=w466, "Value"="Closing all existing VISA devices", "String reference in"=w465) -> ("STring reference out"=w464:refnum<vi>)  [unwired: 8 in]
        n205 = for {
          tunnel: w467 -> [w471] mode=indexing
          shift-right: [w470] -> w462
          shift-left: w466 -> [w472]
          n206 = VISA Close(VISA resource name=w471, error in (no error)=w472) -> (error out=w470:errorcluster)
        }
      }
      frame "Example Finder" {
        n207 = Unbundle By Name(w485) -> ("appended path"=w486:path, "Device type"=w484:string[])
        n208 = call "Find Curriculum.vi"("error in (no error)"=w479, "Array ot connected evices"=w484, "Location of Examples"=w486) -> ("error out"=w474:errorcluster, "Is the required hardware detected?"=w475:bool[], "Example File Paths"=w476:path[])  [unwired: 6 in]
        n209 = Format Into String(format string="Looking for examples at \"%s\"", w486) -> (resulting string=w488:string)  [unwired: 2 in, 1 out]
        n210 = call "Status String Update.vi"("error in (no error)"=w474, "Value"=w488, "String reference in"=w487) -> ("STring reference out"=w483:refnum<vi>)  [unwired: 8 in]
        n211 = Unbundle By Name(w485) -> ("Array of VISA Resources"=w477:refnum<visa-resource-name>[], "Device type"=w478:string[])
        n212 = call "Status String Update.vi"("error in (no error)"=w474, "Value"="Opening Curriculum Launcher " ("format string"), "String reference in"=w483) -> ("STring reference out"=w481:refnum<vi>)  [unwired: 8 in]
        n213 = call "Curriculum Launcher.vi"("Array of VISA Resources"=w477, "Device type"=w478, "error in (no error)"=w474, "Is the required hardware detected?"=w475, "Example File Paths"=w476) -> ("error out"=w473:errorcluster)  [unwired: 6 in]
        n214 = for {
          tunnel: w476 -> [w492] mode=indexing
          tunnel: w475 -> [w497] mode=indexing
          shift-right: [w490] -> w480
          shift-left: w481 -> [w499]
          n215 = Strip Path(path=w492) -> (name=w491:string)  [unwired: 1 out]
          n216 = Select(t="Yes" ("input 2"), s=w497, f="No" ("input 2")) -> (s? t:f=w494:string)
          n217 = Format Into String(format string="Found example \"%s.\" Required hardware present? %s", w491, w494) -> (resulting string=w493:string)  [unwired: 2 in, 1 out]
          n218 = call "Status String Update.vi"("Value"=w493, "String reference in"=w499) -> ("STring reference out"=w490:refnum<vi>)  [unwired: 9 in]
        }
      }
    }
    n219 = call "Status String Update.vi"("error in (no error)"=w113, "Value"=w121, "String reference in"=w118) -> ()  [unwired: 8 in, 1 out]
    n220 = call <vilib>:"Clear Errors.vi"("error in (no error)"=w113) -> ("error out"=w115:errorcluster)  [unwired: 5 in, 1 out]
  }
